vi "Read.vi"(8 "error in (no error)":errorcluster, 11 "HW-201 in":refnum<class "HW-201.lvclass">) -> (0 "error out":errorcluster, 3 "HW-201 out":refnum<class "HW-201.lvclass">)   [LabVIEW 2022 SP3, in "HW-201.lvlib" / "HW-201.lvclass"]
uses:
  HW-201.lvclass
  HW-201.lvclass/HW-201.ctl
  <vilib>/MakerHub/LINX/LMH-LINX.lvlib
  <vilib>/MakerHub/LINX/Public/Peripherals/Digital/Digital Read 1 Chan.vi
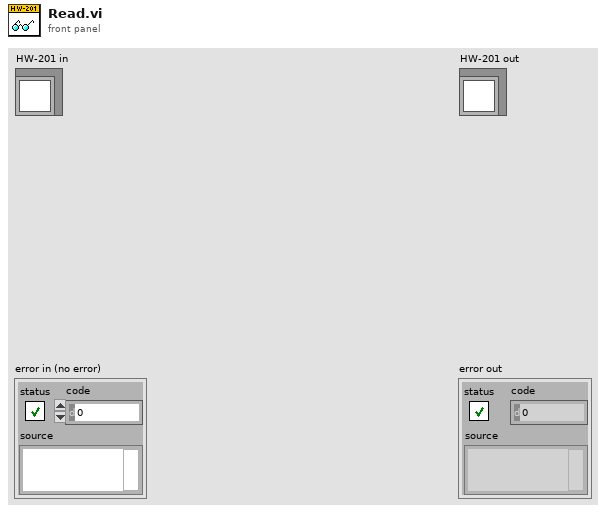
[diagram p1: front panel]
types:
  T1 = typedef "LMH-LINX.lvlib/LINX Ref.ctl" = cluster{"IO":T2, "Interface":T3, "LINX Device Config":T4}
  T2 = typedef "LMH-LINX.lvlib/Platform.ctl" = enum16{"Remote", "Local"}
  T3 = typedef "LMH-LINX.lvlib/Interface.ctl" = enum16{"Serial", "TCP"}
  T4 = typedef "LMH-LINX.lvlib/Device.lvlib/LINX Device Config.ctl" = cluster{"Interface":T3, "COM Port":refnum<visa-resource-name>, "TCP Configuration":T5, "Device Family":u8, "Device ID":u8, "Device Name":string, "TCP Ref":refnum<k5>, "Channels":T6}
  T5 = typedef "LMH-LINX.lvlib/Device.lvlib/TCP Config.ctl" = cluster{"IP Address":string, "Port":u16}
  T6 = typedef "LMH-LINX.lvlib/Channels.ctl" = cluster{"DI":u8[], "DO":u8[], "AI":u8[], "AO":u8[], "PWM":u8[], "QE":u8[], "UART":u8[], "I2C 2":u8[], "SPI":u8[], "CAN":u8[], "Servo":u8[], "AI Ref (V)":dbl, "AI Resolution (Bits)":u8, "AO Ref (V)":dbl, "AO Resolution (Bits)":u8}
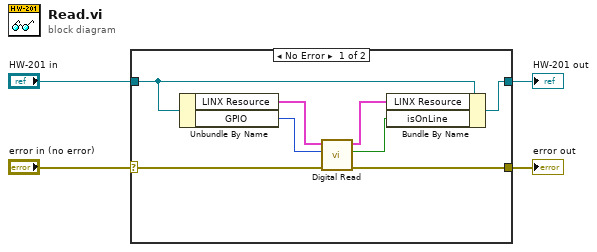
[diagram p0: block diagram]
diagram:
  n1 = case shown="No Error" "error in (no error)" {
    selector: "error in (no error)" -> [w5 w14]
    tunnel: [w11 w14] -> w3
    tunnel: [w10 w13] -> w1
    tunnel: "HW-201 in" -> [w12 w13]
    frame No Error {
      n2 = Unbundle By Name(w12) -> ("LINX Resource"=w6:T1, "GPIO"=w7:u8)
      n3 = call-poly <vilib>:"Digital Read.vi"("Error In"=w5, "DI Channel"=w7, "LINX Resource"=w6) -> ("Error Out"=w11:errorcluster, "DI Value"=w9:bool, "LINX Resource"=w8:T1)  [unwired: 6 in]
      n4 = Bundle By Name(cluster=w12, "LINX Resource"=w8, "isOnLine"=w9) -> (w10:refnum<class "HW-201.lvclass">)
    }
    frame Error {
    }
  }
  "error out" <- w3
  "HW-201 out" <- w1
